vi "Resume Logging.vi"(8 "error in (no error)":errorcluster, 11 "TDMS Data Logger Actor in":refnum<class "TDMS Data Logger Actor.lvclass">) -> (0 "error out":errorcluster, 3 "TDMS Data Logger Actor out":refnum<class "TDMS Data Logger Actor.lvclass">)   [LabVIEW 2024, in "TDMS Data Logger Actor.lvlib" / "TDMS Data Logger Actor.lvclass"]
uses:
  TDMS Data Logger Actor.lvclass
  C:/Program Files (x86)/National Instruments/LabVIEW 2024/vi.lib/ActorFramework/Actor/Actor.lvclass
  TDMS Data Logger Actor.lvclass/TDMS Data Logger Actor.ctl
  <vilib>/ActorFramework/Actor/Actor.lvclass/Actor.ctl
  <vilib>/ActorFramework/Message Enqueuer/Message Enqueuer.lvclass/Message Enqueuer.ctl
  <vilib>/ActorFramework/Message Enqueuer/Enqueue.vi
  Data Logger Actor Reply Interface/Data Logger Actor Reply Interface Messages/Logging Active Msg/Logging Active Msg.lvclass
  C:/Program Files (x86)/National Instruments/LabVIEW 2024/vi.lib/ActorFramework/Message/Message.lvclass
  <vilib>/ActorFramework/Message Priority Queue/Priority Enqueue.vi
  <vilib>/ActorFramework/Actor/Actor.lvclass
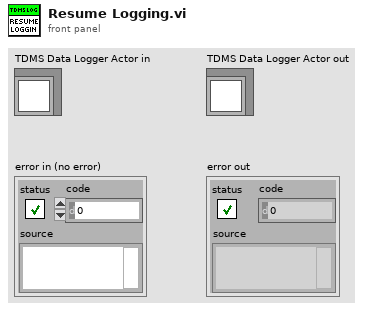
[diagram p1: front panel]
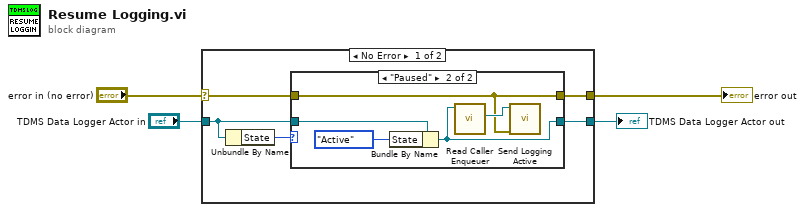
[diagram p0: block diagram]
diagram:
  n1 = case shown="No Error" "error in (no error)" {
    selector: "error in (no error)" -> [w7 w18]
    tunnel: "TDMS Data Logger Actor in" -> [w8 w17]
    tunnel: [w6 w18] -> w2
    tunnel: [w5 w17] -> w1
    frame No Error {
      n2 = Unbundle By Name(w8) -> ("State"=w9:enum16{"Idle", "Active", "Paused"})
      n3 = case shown="\"Paused\"" w9 {
        tunnel: w8 -> [w10 w16]
        tunnel: w7 -> [w11 w12]
        tunnel: [w11 w12] -> w6
        tunnel: [w10 w13] -> w5
        frame "Idle", "Active" {
        }
        frame "Paused" {
          n4 = Bundle By Name(cluster=w16, "State"=enum16{"Idle", "Active", "Paused"}."Active") -> (w13:refnum<class "TDMS Data Logger Actor.lvclass">)
          n5 = call <vilib>:"Read Caller Enqueuer.vi"("Actor"=w13) -> ("Caller Enqueuer"=w14:refnum<class "Message Enqueuer.lvclass">)  [unwired: 10 in]
          n6 = call "Send Logging Active.vi"("error in (no error)"=w12, "Message Enqueuer"=w14) -> ()  [unwired: 8 in, 2 out]
        }
      }
    }
    frame Error {
    }
  }
  "error out" <- w2
  "TDMS Data Logger Actor out" <- w1
